vi "SEA_9811_send_config_to_module.vi"(8 "error in (no error)":errorcluster, 9 "Transmitter Control Register (TCR)":T1={"TCR0: not used"=FALSE, "TCR1: not used"=FALSE, "TCR2: not used"=FALSE, "TCR3: Transmitter Parity Bit Enable: 32nd bit is parity (1) or data (0)"=FALSE, "TCR4: not used"=FALSE, "TCR5: not used"=FALSE, "TCR6: not used"=FALSE, "TCR7: not used"=FALSE, "TCR8: not used"=FALSE, "TCR9: Transmitter Parity Select: odd parity (0) or even parity (1)"=FALSE, "TCR10: Transmitter Data Rate: ARINC 429 high-speed (0) or low-speed (1)"=FALSE, "TCR11: ARINC Label Bit Order: label bit order reversed (0) or not reversed (1)"=FALSE, "TCR12: Disable Line Driver: normal operation (0) or transmitter disabled (1)"=FALSE, "TCR13: Tansmit whenever data is available in FIFO (1) or only start by instruction \"Enable Transmission\" (0)"=TRUE, "TCR14: not used"=FALSE, "TCR15: not used"=FALSE}, 10 "Rx channel":T3, 11 "FPGA Interface Base In":refnum<class "FPGA Interface Base.lvclass">) -> (0 "error out":errorcluster, 3 "FPGA Interface Base Out":refnum<class "FPGA Interface Base.lvclass">)   [LabVIEW 2015]
uses:
  FPGA/SEA-9811_ReceiverAndTransmitter/SubVIs/SEA-9811_ReceiverAndTransmitter_RCR.ctl
  FPGA/SEA-9811_ReceiverAndTransmitter/SubVIs/SEA-9811_ReceiverAndTransmitter_TCR.ctl
  <userlib>/_FPGA Interface Advanced Tools/FPGA Interface Base/FPGA Interface Base.lvclass
  <userlib>/_FPGA Interface Advanced Tools/FPGA Interface Base/FPGA Write By Name - U8.vi
  <userlib>/_FPGA Interface Advanced Tools/FPGA Interface Base/FPGA Write Array By Name - U8.vi
  <userlib>/_FPGA Interface Advanced Tools/FPGA Interface Base/FPGA Write By Name - U16.vi
  <userlib>/_FPGA Interface Advanced Tools/FPGA Interface Base/FPGA Write By Name - Boolean.vi
  <userlib>/_FPGA Interface Advanced Tools/FPGA Interface Base/FPGA Read By Name - Boolean.vi
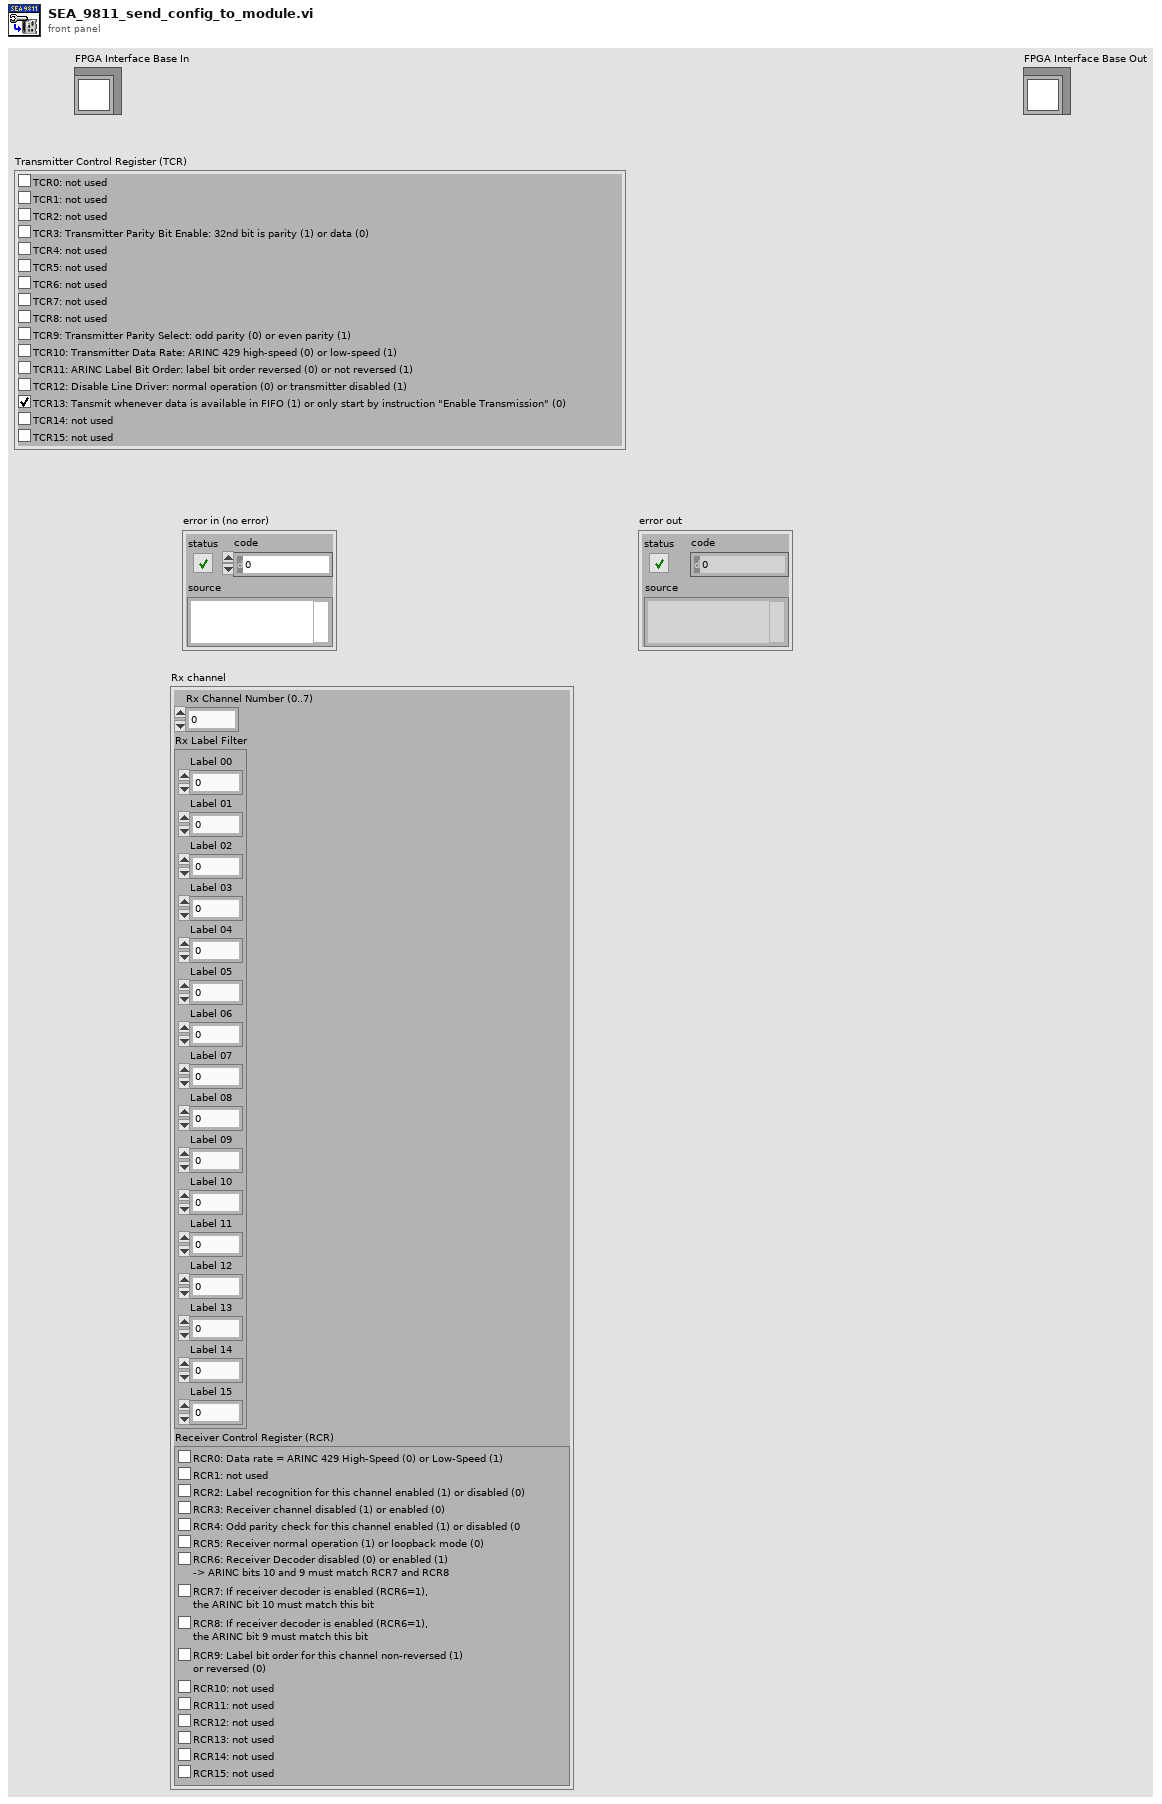
[diagram p1: front panel]
types:
  T1 = typedef "SEA-9811_ReceiverAndTransmitter_TCR.ctl" = cluster{"TCR0: not used":bool, "TCR1: not used":bool, "TCR2: not used":bool, "TCR3: Transmitter Parity Bit Enable: 32nd bit is parity (1) or data (0)":bool, "TCR4: not used":bool, "TCR5: not used":bool, "TCR6: not used":bool, "TCR7: not used":bool, "TCR8: not used":bool, "TCR9: Transmitter Parity Select: odd parity (0) or even parity (1)":bool, "TCR10: Transmitter Data Rate: ARINC 429 high-speed (0) or low-speed (1)":bool, "TCR11: ARINC Label Bit Order: label bit order reversed (0) or not reversed (1)":bool, "TCR12: Disable Line Driver: normal operation (0) or transmitter disabled (1)":bool, "TCR13: Tansmit whenever data is available in FIFO (1) or only start by instruction \"Enable Transmission\" (0)":bool, "TCR14: not used":bool, "TCR15: not used":bool}
  T2 = typedef "SEA-9811_ReceiverAndTransmitter_RCR.ctl" = cluster{"RCR0: Data rate = ARINC 429 High-Speed (0) or Low-Speed (1)":bool, "RCR1: not used":bool, "RCR2: Label recognition for this channel enabled (1) or disabled (0)":bool, "RCR3: Receiver channel disabled (1) or enabled (0)":bool, "RCR4: Odd parity check for this channel enabled (1) or disabled (0":bool, "RCR5: Receiver normal operation (1) or loopback mode (0)":bool, "RCR6: Receiver Decoder disabled (0) or enabled (1) \n-> ARINC bits 10 and 9 must match RCR7 and RCR8":bool, "RCR7: If receiver decoder is enabled (RCR6=1), \nthe ARINC bit 10 must match this bit":bool, "RCR8: If receiver decoder is enabled (RCR6=1), \nthe ARINC bit 9 must match this bit":bool, "RCR9: Label bit order for this channel non-reversed (1) \nor reversed (0)":bool, "RCR10: not used":bool, "RCR11: not used":bool, "RCR12: not used":bool, "RCR13: not used":bool, "RCR14: not used":bool, "RCR15: not used":bool}
  T3 = cluster{"Rx Channel Number (0..7)":u8, "Rx Label Filter":cluster{"Label 00":u8, "Label 01":u8, "Label 02":u8, "Label 03":u8, "Label 04":u8, "Label 05":u8, "Label 06":u8, "Label 07":u8, "Label 08":u8, "Label 09":u8, "Label 10":u8, "Label 11":u8, "Label 12":u8, "Label 13":u8, "Label 14":u8, "Label 15":u8}, "Receiver Control Register (RCR)":T2}
  T4 = cluster{"Label 00":u8, "Label 01":u8, "Label 02":u8, "Label 03":u8, "Label 04":u8, "Label 05":u8, "Label 06":u8, "Label 07":u8, "Label 08":u8, "Label 09":u8, "Label 10":u8, "Label 11":u8, "Label 12":u8, "Label 13":u8, "Label 14":u8, "Label 15":u8}
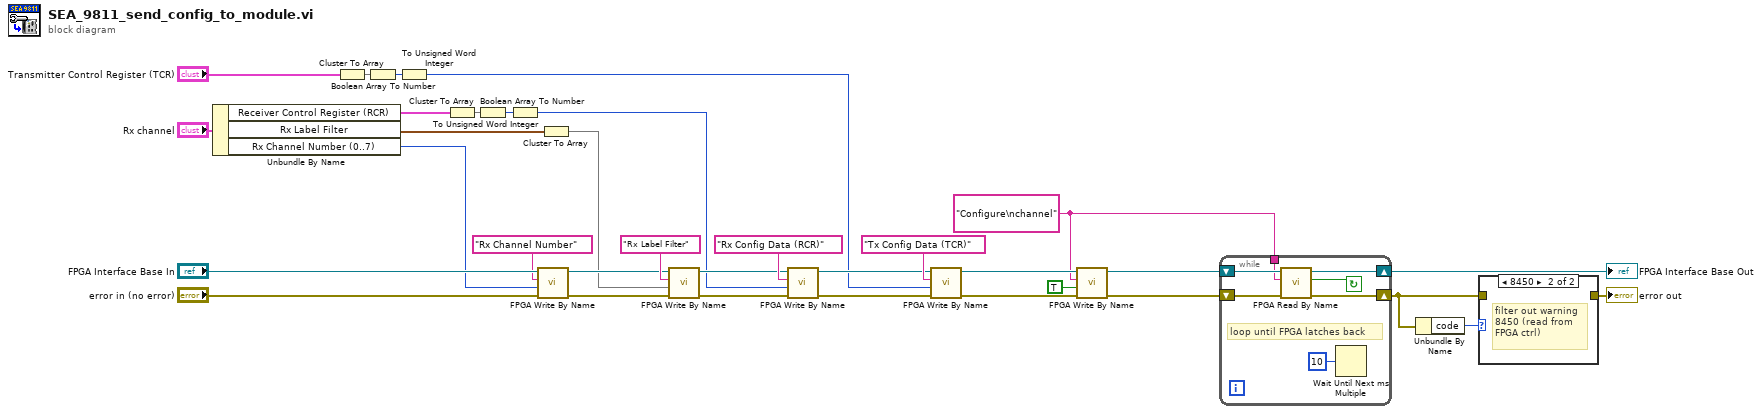
[diagram p0: block diagram]
diagram:
  w4 = "Configure\nchannel" ("Control")
  n1 = Unbundle By Name("Rx channel") -> ("Receiver Control Register (RCR)"=w15:T2, "Rx Label Filter"=w22:T4, "Rx Channel Number (0..7)"=w16:u8)
  n2 = Cluster To Array(cluster="Transmitter Control Register (TCR)") -> (array=w34:bool[])
  n3 = Boolean Array To Number(Boolean array=w34) -> (number=w33:u32)
  n4 = To Unsigned Word Integer(number=w33) -> (unsigned 16bit integer=w11:u16)
  n5 = Cluster To Array(cluster=w15) -> (array=w31:bool[])
  n6 = Boolean Array To Number(Boolean array=w31) -> (number=w32:u32)
  n7 = To Unsigned Word Integer(number=w32) -> (unsigned 16bit integer=w17:u16)
  n8 = call-poly <userlib>:"FPGA Write By Name.vi"("error in (no error)"="error in (no error)", "Value"=w16, "Control"="Rx Channel Number", "FPGA Session In"="FPGA Interface Base In") -> ("error out"=w23:errorcluster, "FPGA Session Out"=w24:refnum<class "FPGA Interface Base.lvclass">)  [unwired: 6 in]
  n9 = Cluster To Array(cluster=w22) -> (array=w21:u8[])
  n10 = call-poly <userlib>:"FPGA Write By Name.vi"("error in (no error)"=w23, "Array"=w21, "Control"="Rx Label Filter", "FPGA Session In"=w24) -> ("error out"=w18:errorcluster, "FPGA Session Out"=w19:refnum<class "FPGA Interface Base.lvclass">)  [unwired: 6 in]
  n11 = call-poly <userlib>:"FPGA Write By Name.vi"("error in (no error)"=w18, "Value"=w17, "Control"="Rx Config Data (RCR)", "FPGA Session In"=w19) -> ("error out"=w12:errorcluster, "FPGA Session Out"=w13:refnum<class "FPGA Interface Base.lvclass">)  [unwired: 6 in]
  n12 = call-poly <userlib>:"FPGA Write By Name.vi"("error in (no error)"=w12, "Value"=w11, "Control"="Tx Config Data (TCR)", "FPGA Session In"=w13) -> ("error out"=w9:errorcluster, "FPGA Session Out"=w10:refnum<class "FPGA Interface Base.lvclass">)  [unwired: 6 in]
  n13 = call-poly <userlib>:"FPGA Write By Name.vi"("error in (no error)"=w9, "Value"=TRUE, "Control"=w4, "FPGA Session In"=w10) -> ("error out"=w7:errorcluster, "FPGA Session Out"=w6:refnum<class "FPGA Interface Base.lvclass">)  [unwired: 6 in]
  n14 = while {
    shift-right: [w38] -> w2
    shift-left: w7 -> [w39]
    shift-right: [w36] -> w5
    shift-left: w6 -> [w37]
    tunnel: w4 -> [w35]
    stop <- w40 continue-if-true
    # "loop until FPGA latches back"
    n15 = call-poly <userlib>:"FPGA Read By Name.vi"("error in (no error)"=w39, "Indicator"=w35, "FPGA Session In"=w37) -> ("error out"=w38:errorcluster, "Value"=w40:bool, "FPGA Session Out"=w36:refnum<class "FPGA Interface Base.lvclass">)  [unwired: 6 in]
    n16 = Wait Until Next ms Multiple(millisecond multiple=u32 10) -> ()  [unwired: 1 out]
  }
  "FPGA Interface Base Out" <- w5
  n17 = Unbundle By Name(w2) -> ("code"=w3:i32)
  n18 = case shown="8450" w3 {
    tunnel: w2 -> [w42 _]
    tunnel: [w42 _] -> w1
    frame 0, Default {
    }
    frame 8450 {
      # "filter out warning\n8450 (read from\nFPGA ctrl)"
    }
  }
  "error out" <- w1
